vi "SignalGenerator_fxp16.vi"(10 "phase":fxp<+,64,64>, 11 "Reset":bool) -> (0 "data_valid":bool, 1 "Cos":fxp<+/-,16,0>, 2 "Sin":fxp<+/-,16,0>)   [LabVIEW 2025]
uses:
  <vilib>/rvi/XilinxIP/XIPIN_XNode/niFpgaXIPIN.xnode
  <vilib>/rvi/FXPMathLib/FxpInterpret/XNode/nifxpmath_Interpret.xnode
  FPGA/Filters/SignalGenerator/DDS Compiler/xsim.dir/DDS_Compiler_6207C7FBB7E34A25803D623AF424DDD8/xsimk_6207C7FBB7E34A25803D623AF424DDD8.dll
  <vilib>/rvi/IPIntegrationNode/IPINode_Xnode/niFpgaIPINode.xnode
  <vilib>/rvi/IPIntegrationNode/IPINode_Typedef/niFpgaIPINodeSupportedFamilies.ctl
  <vilib>/rvi/IPIntegrationNode/IPINode_Utilities/niFpgaIPINodeSimCore.vi
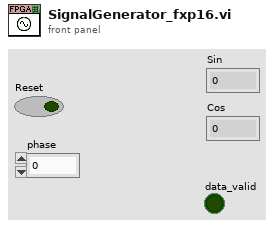
[diagram p1: front panel]
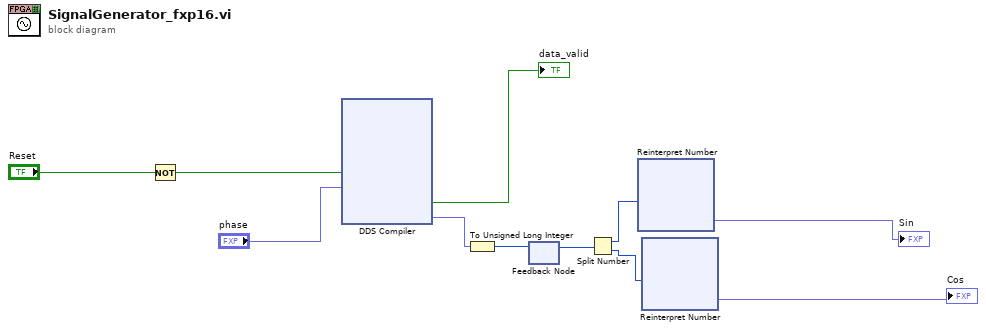
[diagram p0: block diagram]
diagram:
  n1 = Not(x="Reset") -> (.not. x?=w4:bool)
  n2 = xnode ("DDS Compiler")("aresetn"=w4, "s_axis_phase_tdata"="phase") -> ("m_axis_data_tvalid"=→"data_valid":bool, "m_axis_data_tdata"=w1:fxp<+,32,32>)  [unwired: 2 in]
  n3 = To Unsigned Long Integer(number=w1) -> (unsigned 32bit integer=w6:u32)
  n4 = feedback #1() -> (w5:u32)  [unwired: 1 in]
  n5 = feedback-in #1(w6) -> ()
  n6 = Split Number(x=w5) -> (hi(x)=w11:u16, lo(x)=w10:u16)
  n7 = xnode "Reinterpret Number"("x"=w11) -> ("y"=→"Sin":fxp<+/-,16,0>)
  n8 = xnode "Reinterpret Number"("x"=w10) -> ("y"=→"Cos":fxp<+/-,16,0>)
